vi "pwm set.vi"(8 "error in":errorcluster, 9 "motor  ?":enum16{"M1", "M2", "M3", "M4"}(ring), 10 "PWM":cluster{"divider":i32, "period":i32}, 11 "FPGA VI Reference In":refnum<k20>) -> (0 "error out":errorcluster, 3 "FPGA VI Reference Out":refnum<k20>)   [LabVIEW 2019, in "my FPGA lib.lvlib" / "motor.lvclass"]
uses:
  motor.lvclass
  <vilib>/Utility/error.llb/Error Cluster From Error Code.vi
  <vilib>/rvi/errors/niLvFpgaAdjustHostInterfaceError.vi
  <vilib>/rvi/interface/nirviReadWriteControl/nirviReadWriteControl.xnode
  NiFpgaLv.dll
  <vilib>/rvi/interface/Simulation/niFpgaSimulationCallBeginRW.vi
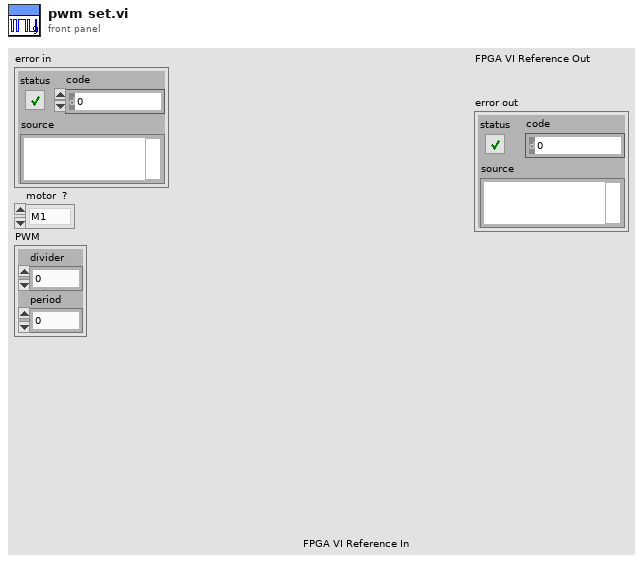
[diagram p1: front panel]
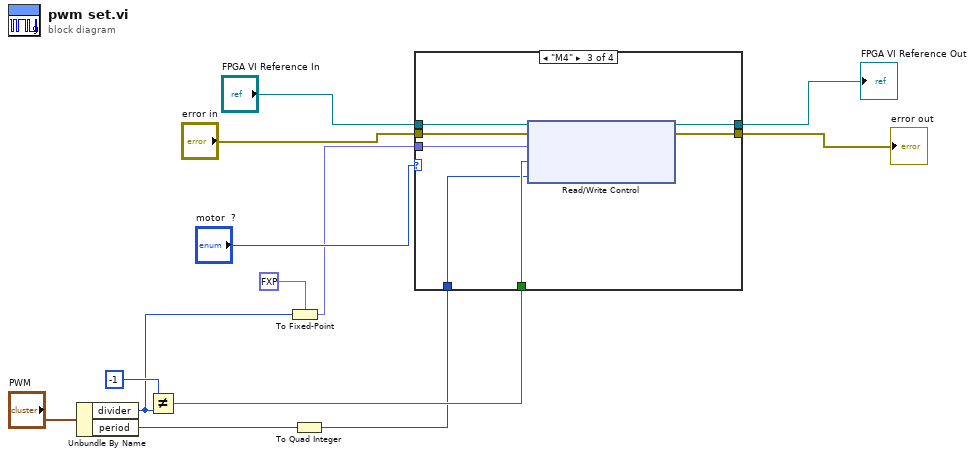
[diagram p0: block diagram]
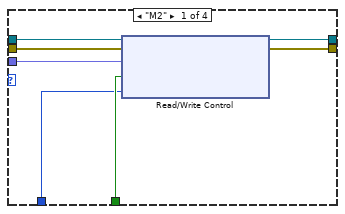
[diagram p2: hidden frame]
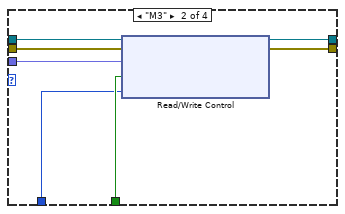
[diagram p3: hidden frame]
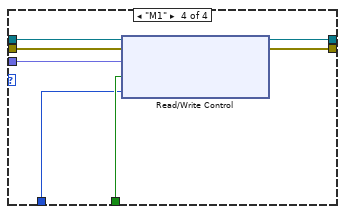
[diagram p4: hidden frame]
diagram:
  n1 = Unbundle By Name("PWM") -> ("divider"=w5:i32, "period"=w7:i32)
  n2 = Not Equal?(x=-1, y=w5) -> (x != y?=w8:bool)
  n3 = To Fixed-Point(fixed-point type=fxp<+,4,4> 0.0, number=w5) -> (fixed-point=w4:fxp<+,4,4>)
  n4 = To Quad Integer(1:w7) -> (0:w6:i64)
  n5 = case shown="\"M4\"" "motor  ?" {
    tunnel: "FPGA VI Reference In" -> [w20 w27 w34 w41]
    tunnel: "error in" -> [w19 w26 w33 w40]
    tunnel: w8 -> [w17 w24 w32 w38]
    tunnel: w6 -> [w16 w23 w31 w37]
    tunnel: w4 -> [w18 w25 w30 w39]
    tunnel: [w14 w21 w28 w36] -> w1
    tunnel: [w15 w22 w29 w35] -> w2
    frame "M2" {
      n6 = xnode "Read/Write Control"("FPGA VI Reference In"=w20, "error in"=w19, "Motor2.divider"=w18, "Motor2.enable_divider"=w17, "Motor2.periode"=w16) -> ("FPGA VI Reference Out"=w15:refnum<k20>, "error out"=w14:errorcluster)
    }
    frame "M3" {
      n7 = xnode "Read/Write Control"("FPGA VI Reference In"=w27, "error in"=w26, "Motor3.divider"=w25, "Motor3.enable_divider"=w24, "Motor3.periode"=w23) -> ("FPGA VI Reference Out"=w22:refnum<k20>, "error out"=w21:errorcluster)
    }
    frame "M4" {
      n8 = xnode "Read/Write Control"("FPGA VI Reference In"=w34, "error in"=w33, "Motor4.divider"=w30, "Motor4.enable_divider"=w32, "Motor4.periode"=w31) -> ("FPGA VI Reference Out"=w29:refnum<k20>, "error out"=w28:errorcluster)
    }
    frame "M1" {
      n9 = xnode "Read/Write Control"("FPGA VI Reference In"=w41, "error in"=w40, "Motor1.divider"=w39, "Motor1.enable_divider"=w38, "Motor1.periode"=w37) -> ("FPGA VI Reference Out"=w35:refnum<k20>, "error out"=w36:errorcluster)
    }
  }
  "FPGA VI Reference Out" <- w2
  "error out" <- w1
